vi "RisingEdgeTrigger.vi"(1 "Raw Signal":bool) -> (0 "Trigger":bool)   [LabVIEW 2019]
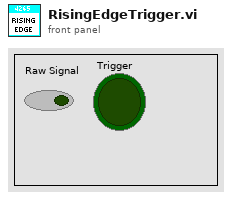
[diagram p1: front panel]
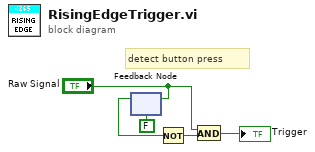
[diagram p0: block diagram]
diagram:
  # "detect button press"
  n1 = feedback #1(FALSE ("Button")) -> (w3:bool)
  n2 = feedback-in #1("Raw Signal") -> ()
  n3 = Not(x=w3) -> (.not. x?=w5:bool)
  n4 = And(x="Raw Signal", y=w5) -> (x .and. y?=→"Trigger":bool)
